vi "sv_Log View for Band Power (1 Ch).vi"(0 "octave spectrum":T6 {"band power [EU^2 rms]" format="%.2f"; "nominal frequencies [Hz]" format="%.2f"}, 9 "octave info":T1={"standard"=enum."ANSI S1.11", "bandwidth"=enum."1 octave", "low band"=0, "high band"=0, "weighting filter"=0, "dB reference"=0.0, "dB On"=FALSE, "unit label"="", "channel name"="", "description"="", "engineering units"=1, "custom label"="", "spectrum type"=enum."magnitude", "spectral density"=FALSE, "filters settled"=FALSE} {"engineering units" items=["custom..."=0, "V"=1, "A"=21, "C"=30, "pC"=31, "s"=32, "-"=29, "Pa"=2, "N"=20, "g"=3, "m/s^2"=4, "m/s"=5, "m"=6, "mm/s"=12, "mm"=13, "micron/s"=14, "micron"=15, "in/s^2"=7, "in/s"=8, "in"=9, "mil/s"=10, "mil"=11, "rad/s^2"=16, "rad/s"=17, "rad"=18, "deg/s^2"=26, "deg/s"=27, "deg"=28, "RPM"=22, "cycle/s^2"=23, "Hz"=24, "cycle"=25, "strain"=19]; "dB reference" format="%.2e"; "weighting filter" items=["Linear", "A-weighting", "B-weighting", "C-weighting", "ITU-R 468-4", "Dolby", "CCITT", "C-message", "Wb", "Wc", "Wd", "We", "Wf", "Wh", "Wj", "Wk", "Wm", "AES17 20 kHz lowpass", "AES17 40 kHz lowpass", "AES17 20 kHz highpass", "AES17 40 kHz highpass"]}, 11 "error in (no error)":errorcluster, 12 "dB On (T)":bool=TRUE) -> (4 "octave spectrum":T5 {"band power [dB EU]" format="%.2f"; "nominal frequencies [Hz]" format="%.2f"}, 6 "unit label":string, 10 "octave info":T1={"standard"=enum."ANSI S1.11", "bandwidth"=enum."1 octave", "low band"=0, "high band"=0, "weighting filter"=0, "dB reference"=0.0, "dB On"=FALSE, "unit label"="", "channel name"="", "description"="", "engineering units"=1, "custom label"="", "spectrum type"=enum."magnitude", "spectral density"=FALSE, "filters settled"=FALSE} {"engineering units" items=["custom..."=0, "V"=1, "A"=21, "C"=30, "pC"=31, "s"=32, "-"=29, "Pa"=2, "N"=20, "g"=3, "m/s^2"=4, "m/s"=5, "m"=6, "mm/s"=12, "mm"=13, "micron/s"=14, "micron"=15, "in/s^2"=7, "in/s"=8, "in"=9, "mil/s"=10, "mil"=11, "rad/s^2"=16, "rad/s"=17, "rad"=18, "deg/s^2"=26, "deg/s"=27, "deg"=28, "RPM"=22, "cycle/s^2"=23, "Hz"=24, "cycle"=25, "strain"=19]; "dB reference" format="%.2e"; "weighting filter" items=["Linear", "A-weighting", "B-weighting", "C-weighting", "ITU-R 468-4", "Dolby", "CCITT", "C-message", "Wb", "Wc", "Wd", "We", "Wf", "Wh", "Wj", "Wk", "Wm", "AES17 20 kHz lowpass", "AES17 40 kHz lowpass", "AES17 20 kHz highpass", "AES17 40 kHz highpass"]}, 14 "total band power [dB EU]":dbl format="%.2f", 15 "error out":errorcluster)   [LabVIEW 2017, in "SoundVib_Octave_2014 standard.lvlib"]
uses:
  <vilib>/addons/Sound and Vibration/svt_Octave/SoundVib_Octave_2014 standard.lvlib
  <vilib>/addons/_NISVFA/_Shared subVIs/Controls/svc_Octave Info.ctl
  <vilib>/addons/_NISVFA/_Shared subVIs/Controls/svc_Octave Standard.ctl
  <vilib>/addons/_NISVFA/_Shared subVIs/Controls/svc_Weighting Filter Text Ring.ctl
  <vilib>/addons/_NISVFA/_Shared subVIs/Controls/svc_Engineering Units Text Ring.ctl
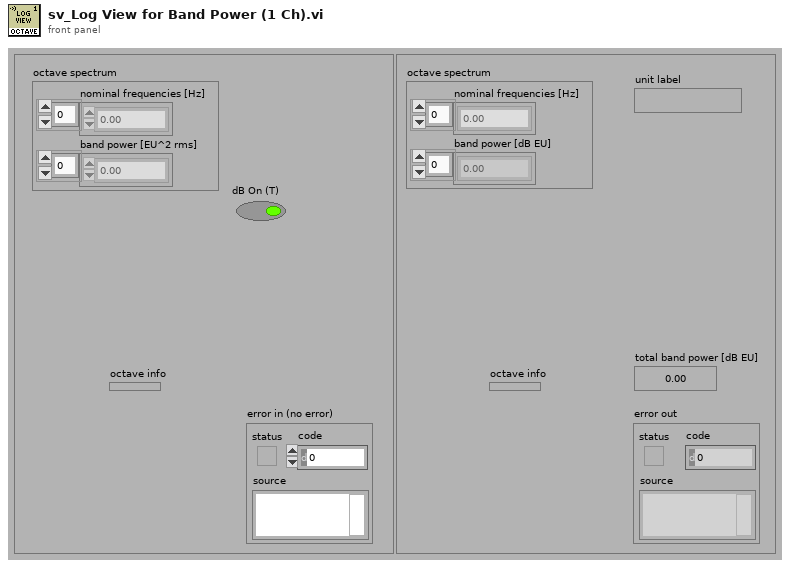
[diagram p1: front panel]
types:
  T1 = typedef "svc_Octave Info.ctl" = cluster{"standard":T2, "bandwidth":enum16{"1 octave", "1/3 octave", "1/6 octave", "1/12 octave", "1/24 octave"}, "low band":i32, "high band":i32, "weighting filter":T3, "dB reference":dbl, "dB On":bool, "unit label":string, "channel name":string, "description":string, "engineering units":T4, "custom label":string, "spectrum type":enum16{"power", "magnitude"}, "spectral density":bool, "filters settled":bool}
  T2 = typedef "svc_Octave Standard.ctl" = enum16{"ANSI S1.11", "IEC 61260"}
  T3 = typedef "svc_Weighting Filter Text Ring.ctl" = u16
  T4 = typedef "svc_Engineering Units Text Ring.ctl" = u16
  T5 = cluster{"nominal frequencies [Hz]":dbl[], "band power [dB EU]":dbl[]}
  T6 = cluster{"nominal frequencies [Hz]":dbl[], "band power [EU^2 rms]":dbl[]}
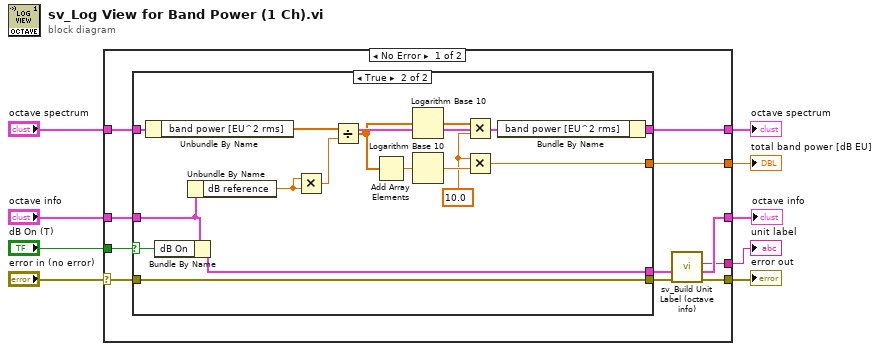
[diagram p0: block diagram]
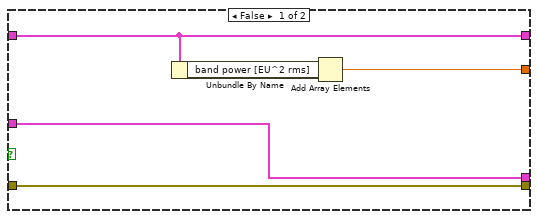
[diagram p2: hidden frame]
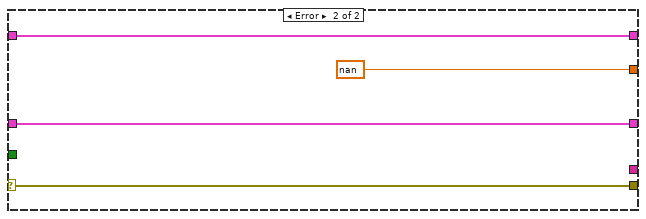
[diagram p3: hidden frame]
diagram:
  n1 = case shown="No Error" "error in (no error)" {
    selector: "error in (no error)" -> [w15 w44]
    tunnel: "dB On (T)" -> [w20 _]
    tunnel: [w13 w44] -> w9
    tunnel: [w19 nan] -> w8
    tunnel: [w10 _] -> w7
    tunnel: "octave spectrum" -> [w18 w43]
    tunnel: [w17 w43] -> w4
    tunnel: "octave info" -> [w16 w42]
    tunnel: [w11 w42] -> w2
    frame No Error {
      n2 = case shown="True" w20 {
        selector: w20 -> [_ w37]
        tunnel: [w23 w30] -> w17
        tunnel: w18 -> [w23 w31]
        tunnel: [w21 w38] -> w19
        tunnel: w15 -> [w25 w36]
        tunnel: [w25 w36] -> w14
        tunnel: w16 -> [w24 w35]
        tunnel: [w24 w28] -> w12
        frame False {
          n3 = Unbundle By Name(w23) -> ("band power [EU^2 rms]"=w22:dbl[])
          n4 = Add Array Elements(numeric array=w22) -> (sum=w21:dbl)
        }
        frame True {
          w39 = 10.0 ("y")
          n5 = Unbundle By Name(w31) -> ("band power [EU^2 rms]"=w32:dbl[])
          n6 = Bundle By Name(cluster=w35, "dB On"=w37) -> (w28:T1)
          n7 = Unbundle By Name(w35) -> ("dB reference"=w34:dbl)
          n8 = Multiply(x=w34, y=w34) -> (x*y=w33:dbl)
          n9 = Divide(x=w32, y=w33) -> (x/y=w27:dbl[])
          n10 = Add Array Elements(numeric array=w27) -> (sum=w26:dbl)
          n11 = Logarithm Base 10(1:w27) -> (0:w41:dbl[])
          n12 = Logarithm Base 10(1:w26) -> (0:w40:dbl)
          n13 = Multiply(x=w41, y=w39) -> (x*y=w29:dbl[])
          n14 = Multiply(x=w39, y=w40) -> (x*y=w38:dbl)
          n15 = Bundle By Name(cluster=w31, "band power [EU^2 rms]"=w29) -> (w30:T6)
        }
      }
      n16 = call <vilib>:"sv_Build Unit Label (octave info).vi"("error in (no error)"=w14, "octave info"=w12) -> ("error out"=w13:errorcluster, "octave info out"=w11:T1, "unit label"=w10:string)  [unwired: 7 in]
    }
    frame Error {
    }
  }
  "error out" <- w9
  "total band power [dB EU]" <- w8
  "unit label" <- w7
  "octave spectrum" <- w4
  "octave info" <- w2
